vi "RT Driver_Compute Correction.vi"(8 "error in (no error)":errorcluster, 10 "Synchronization Interval":dbl, 11 "Offset (s)":dbl format="%_4p") -> (0 "error out":errorcluster, 3 "Correction (S/s)":dbl format="%_4p")   [LabVIEW 2013, in "SNTP Light Custom Device Engine.lvlib"]
doc: "This VI is used to compute correction to apply. \nIf Offset is in the [-0.001; 0.001] second range, we don't apply a correction."
uses:
  SNTP Light Custom Device Engine.lvlib
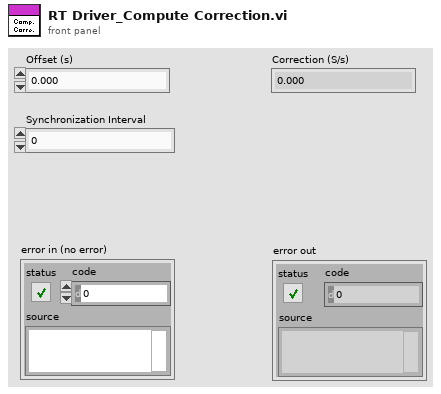
[diagram p1: front panel]
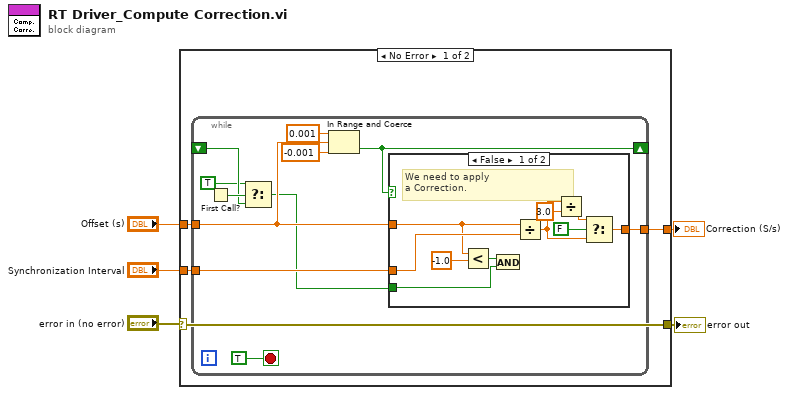
[diagram p0: block diagram]
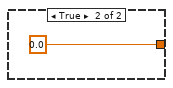
[diagram p2: hidden frame]
diagram:
  n1 = case shown="No Error" "error in (no error)" {
    selector: "error in (no error)" -> [w9 w32]
    tunnel: [w9 w32] -> w4
    tunnel: "Synchronization Interval" -> [w8 _]
    tunnel: "Offset (s)" -> [w6 _]
    tunnel: [w7 _] -> w1
    frame No Error {
      n2 = while {
        tunnel: w8 -> [w20]
        tunnel: [w19] -> w7
        tunnel: w6 -> [w18]
        shift-right: [w10] -> _
        shift-left: _ -> [w13]
        stop <- TRUE stop-if-true
        n3 = First Call?() -> (First Call?: T/F=w14:bool)
        n4 = Select(t=TRUE, s=w14, f=w13) -> (s? t:f=w11:bool)
        n5 = In Range and Coerce(upper limit=0.001, x=w18, lower limit=-0.001) -> (In Range?=w10:bool)  [unwired: 1 out]
        n6 = case shown="False" w10 {
          tunnel: w20 -> [w30 _]
          tunnel: [w25 0.0] -> w19
          tunnel: w18 -> [w29 _]
          tunnel: w11 -> [w26 _]
          frame False {
            # "We need to apply\na Correction."
            n7 = Less?(x=w29, y=-1.0) -> (x < y?=w27:bool)
            n8 = And(x=w27, y=w26) -> ()  [unwired: 1 out]
            n9 = Divide(x=w29, y=w30) -> (x/y=w23:dbl)
            n10 = Divide(x=w23, y=3.0) -> (x/y=w24:dbl)
            n11 = Select(t=w24, s=FALSE, f=w23) -> (s? t:f=w25:dbl)
          }
          frame True {
          }
        }
      }
    }
    frame Error {
    }
  }
  "Correction (S/s)" <- w1
  "error out" <- w4
